vi "ROI entry-User ROI event-Analyse.vi"(8 "error in (no error)":errorcluster, 11 "Event Type":u32) -> (0 "error out":errorcluster, 2 "output cluster":T2 {"ROIs Info []"."FOV" min=1.0 max=10.0 step=1.0; "ROIs Info []"."Frame Size" min=1.0 max=10.0 step=1.0; "ROIs Info []"."Laser Power" min=1.0 max=10.0 step=0.10000000149011612; "ROIs Info []"."Rel. Resolution" min=1.0 max=10.0 step=1.0; "ROIs Info []"."POI Dwell time" min=1.0 max=10.0 step=0.10000000149011612; "ROIs Info []"."Zoom" min=1.0 max=10.0 step=0.10000000149011612; "Last Image Display Event info"."Tool" items=["None", "Selection Tool", "Point Tool", "Line Tool", "Rectangle Tool", "Oval Tool", "Polygon Tool", "ClosedFreehandTool", "Annulus Tool", "Rotated Rectangle Tool", "Zoom Tool", "Pan Tool", "Polyline Tool", "Freehand Tool"]; "Last Image Display Event info"."Type" items=["No Event"=0, "Click Event"=1, "Draw Event"=2, "Size Event"=4, "Scroll Event"=5, "Double Click Event"=8]})   [LabVIEW 2020]
uses:
  Typedefs/ROI Entry screen VI interface 1.ctl
  Typedefs/Last Image Display Event info.ctl
  Typedefs/ROI spec.ctl
  Typedefs/ROI ID Enum.ctl
  Typedefs/ROI info cluster.ctl
  ROI Entry screen/Globals/gl_ROI Entry UI globals.vi
panel:
  out "ROI info cluster (native format)":T1
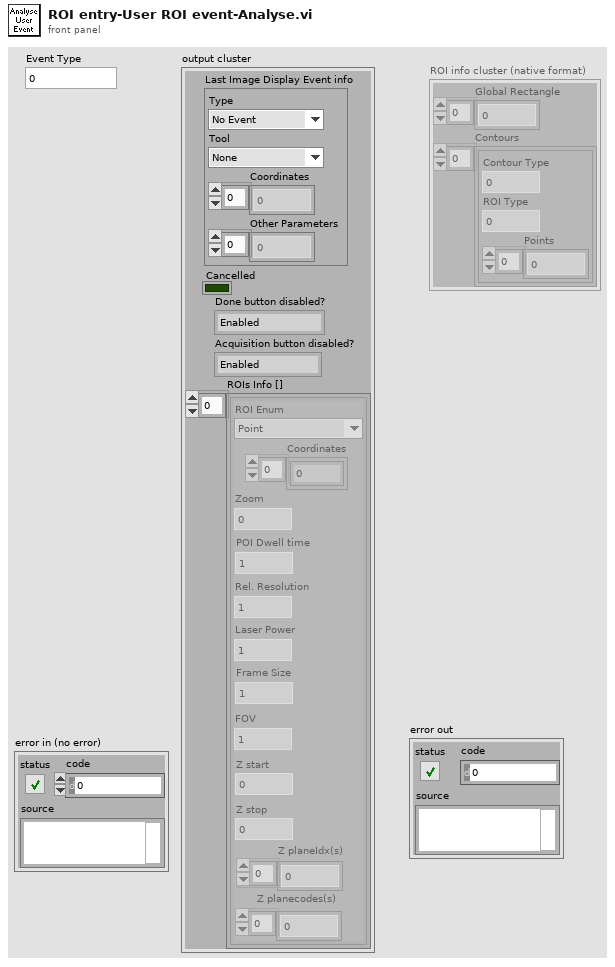
[diagram p1: front panel]
types:
  T1 = typedef "ROI info cluster.ctl" = cluster{"Global Rectangle":i32[], "Contours":cluster{"Contour Type":u32, "ROI Type":u32, "Points":i32[]}[]}
  T2 = typedef "ROI Entry screen VI interface 1.ctl" = cluster{"Last Image Display Event info":T3, "ROIs Info []":T4[], "Cancelled":bool, "Done button disabled?":enum8{"Enabled", "Disabled", "Disabled and Grayed Out"}, "Acquisition button disabled?":enum8{"Enabled", "Disabled", "Disabled and Grayed Out"}}
  T3 = typedef "Last Image Display Event info.ctl" = cluster{"Type":i32, "Tool":i32, "Coordinates":i32[], "Other Parameters":sgl[]}
  T4 = typedef "ROI spec.ctl" = cluster{"ROI Enum":T5, "Coordinates":i32[], "Zoom":dbl, "POI Dwell time":dbl, "Rel. Resolution":dbl, "Laser Power":dbl, "Frame Size":dbl, "FOV":dbl, "Z start":dbl, "Z stop":dbl, "Z planeIdx(s)":i32[], "Z planecodes(s)":u8[]}
  T5 = typedef "ROI ID Enum.ctl" = enum16{"Point", "MiniScan", "Comp. MiniScan", "Rectangle", "Comp. volume", "Arb. plane point", "None"}
  T6 = typedef "ROI entry screen ctrl refs cluster.ctl" = cluster{"Done button":refnum<vi>, "Imaging button":refnum<vi>, "Acquisition button":refnum<vi>, "Scan dwell time per pixel (us)":refnum<vi>, "# of planes":refnum<vi>, "Zoom Ctrl":refnum<vi>, "Equal size":refnum<vi>, "Channel":refnum<vi>, "Image Display":refnum<vi>, "Z-Plane Selector":refnum<vi>, "Number of lines left":refnum<vi>, "Z-stack folder path":refnum<vi>, "POI Density":refnum<vi>, "Arb Plane Entry":refnum<vi>, "Whole Plane":refnum<vi>, "Line Mode":refnum<vi>, "Clear Last":refnum<vi>, "Clear All":refnum<vi>, "Delete Lines":refnum<vi>, "Trial Length (sec)":refnum<vi>, "Palette Type":refnum<vi>, "Intensity slider":refnum<vi>, "# POI":refnum<vi>, "Max Z Proj":refnum<vi>, "Zplane ind":refnum<vi>, "Wavelength (nm)":refnum<vi>, "Number of Trials":refnum<vi>, "Funct stim.trig.enable":refnum<vi>, "Funct stim.trig.delay (s)":refnum<vi>, "Line Mode":refnum<vi>, "Step size (µm)":refnum<vi>, "ROI move mode":refnum<vi>, "Cool-down time (s)":refnum<vi>, "Enable cool-down time":refnum<vi>, "Motor Z ind. (um)":refnum<vi>, "AOL Z ind. (um)":refnum<vi>, "Load Reference Image":refnum<vi>, "Rel.  Res.":refnum<vi>, "ROI LIST":refnum<vi>, "Show All":refnum<vi>, "ROI Type":refnum<vi>, "Start Plane":refnum<vi>, "Stop Plane":refnum<vi>, "Offset ROI":refnum<vi>, "Tab Control":refnum<vi>, "Laser Power(%)":refnum<vi>, "Cycle rate":refnum<vi>, "FOV (Ind.)":refnum<vi>, "Frame Size (Ind.)":refnum<vi>, "Resolution (Ind.)":refnum<vi>, "Pixel Density (Ind)":refnum<vi>, "Laser Power (Ind.)":refnum<vi>, "Dwell Time (Ind.)":refnum<vi>, "Adj MC":refnum<vi>}
  T7 = enum8{"Enabled", "Disabled", "Disabled and Grayed Out"}
  T8 = typedef "ROI Z-stack settings info.ctl" = cluster{"Zoom":dbl, "POI Dwell time":dbl, "Rel. Res":dbl, "Laser Power %":dbl, "Frame Size":dbl, "FOV":dbl}
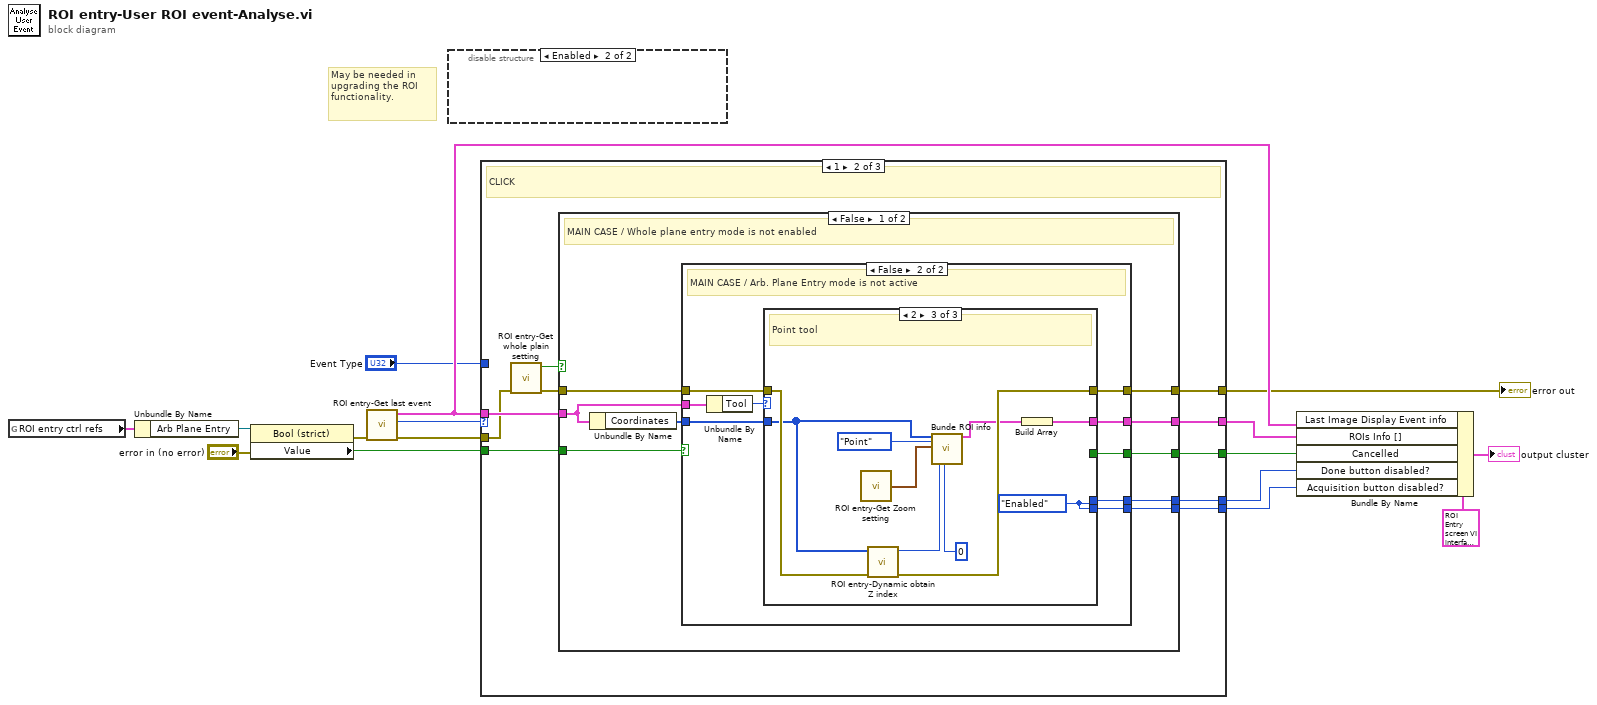
[diagram p0: block diagram]
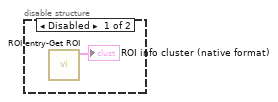
[diagram p2: hidden frame]
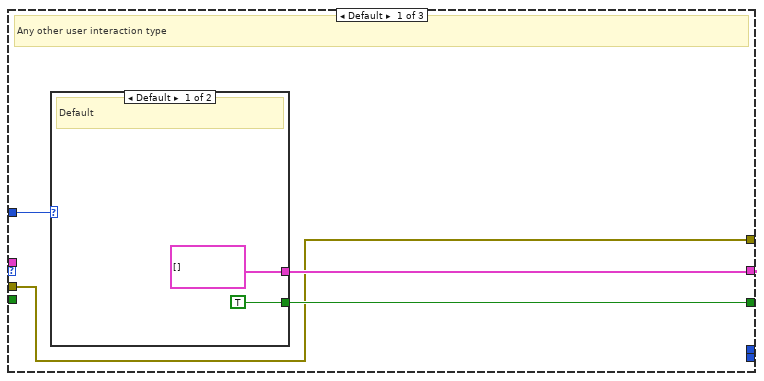
[diagram p3: hidden frame]
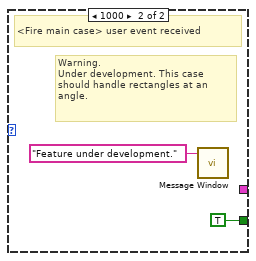
[diagram p4: hidden frame]
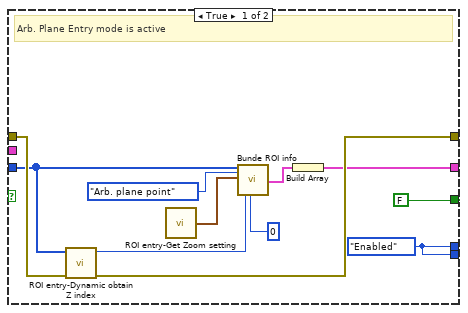
[diagram p5: hidden frame]
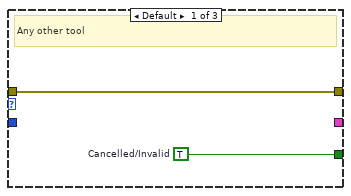
[diagram p6: hidden frame]
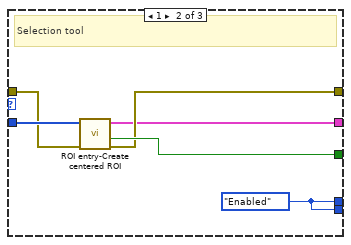
[diagram p7: hidden frame]
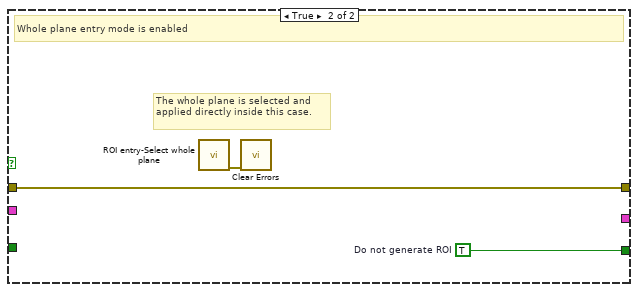
[diagram p8: hidden frame]
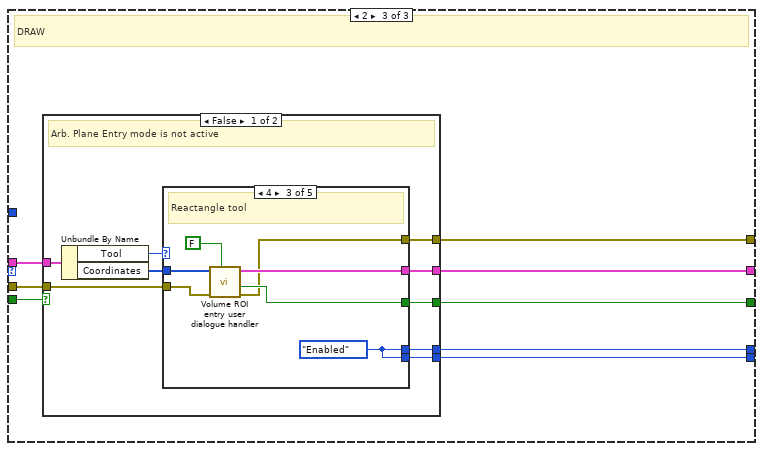
[diagram p9: hidden frame]
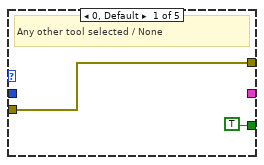
[diagram p10: hidden frame]
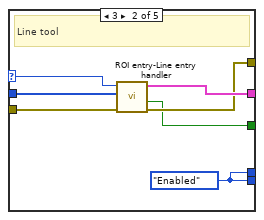
[diagram p11: hidden frame]
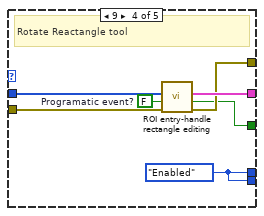
[diagram p12: hidden frame]
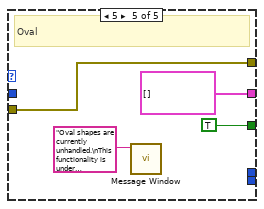
[diagram p13: hidden frame]
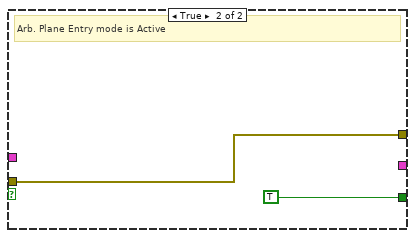
[diagram p14: hidden frame]
diagram:
  # "May be needed in upgrading the ROI functionality."
  n1 = global read "gl_ROI Entry UI globals.vi" "ROI entry ctrl refs"() -> (w15:T6)
  n2 = Unbundle By Name(w15) -> ("Arb Plane Entry"=w14:refnum<vi>)
  n3 = property class="Bool (strict)"(reference=w14, error in="error in (no error)") -> (error out=w4:errorcluster, "Value"=w16:bool)  [unwired: 1 out]
  n4 = call "ROI entry-Get last event.vi"("error in (no error)"=w4) -> ("error out"=w2:errorcluster, "Type"=w6:i32, "Last Image Display Event info"=w13:T3)  [unwired: 8 in]
  n5 = disable-structure shown="Enabled" {
    frame Disabled {
      n6 = call "ROI entry-Get ROI.vi"() -> ("ROI info cluster (native format)"=→"ROI info cluster (native format)":T1)  [unwired: 10 in, 1 out]
    }
    frame Enabled {
    }
  }
  n7 = case shown="1" w6 {
    tunnel: [w20 w26 w93] -> w7
    tunnel: [w19 w35 w92] -> w11
    tunnel: [_ w34 w91] -> w8
    tunnel: [_ w33 w90] -> w9
    tunnel: "Event Type" -> [w21 _ _]
    tunnel: w16 -> [_ w32 w89]
    tunnel: w13 -> [_ w31 w88]
    tunnel: w2 -> [w18 w29 w86]
    tunnel: [w18 w27 w87] -> w1
    frame Default {
      # "Any other user interaction type"
      n8 = case shown="Default" w21 {
        tunnel: [T4[] [] ("ROIs Info []") _] -> w20
        tunnel: [TRUE TRUE ("Cancelled")] -> w19
        frame Default {
          # "Default"
        }
        frame 1000 {
          # "Warning.\nUnder development. This case should handle rectangles at an angle."
          # "<Fire main case> user event received"
          n9 = call "Message Window.vi"("Message string"="Feature under development." ("message")) -> ()  [unwired: 10 in, 1 out]
        }
      }
    }
    frame 1 {
      # "CLICK"
      n10 = call "ROI entry-Get whole plain setting.vi"("error in (no error)"=w29) -> ("error out"=w28:errorcluster, "\"Whole plain?\" value"=w30:bool)  [unwired: 9 in]
      n11 = case shown="False" w30 {
        tunnel: [w44 w85] -> w35
        tunnel: [w43 _] -> w34
        tunnel: [w42 _] -> w33
        tunnel: w32 -> [w41 _]
        tunnel: w31 -> [w39 _]
        tunnel: w28 -> [w36 w83]
        tunnel: [w37 w83] -> w27
        tunnel: [w38 _] -> w26
        frame False {
          # "MAIN CASE / Whole plane entry mode is not enabled"
          n12 = Unbundle By Name(w39) -> ("Coordinates"=w40:i32[])
          n13 = case shown="False" w41 {
            tunnel: w40 -> [w51 w64]
            tunnel: [FALSE ("Do not generate ROI") w63] -> w44
            tunnel: [w55 w62] -> w43
            tunnel: [w55 w61] -> w42
            tunnel: w39 -> [_ w60]
            tunnel: w36 -> [w53 w58]
            tunnel: [w52 w57] -> w37
            tunnel: [w50 w56] -> w38
            frame True {
              w55 = T7."Enabled" ("Disabled")
              # "Arb. Plane Entry mode is active"
              n14 = call "ROI entry-Dynamic obtain Z index.vi"("error in (no error)"=w53, "Coordinates"=w51) -> ("error out"=w52:errorcluster, "Z-plane selector (index)"=w47:i32)  [unwired: 8 in]
              n15 = call "ROI entry-Get Zoom setting.vi"() -> ("AOLZ Settings"=w45:T8)  [unwired: 7 in, 8 out]
              n16 = call "Bunde ROI info.vi"("ROI Coordinates"=w51, "ROI Enum"=ROI_ID_Enum."Arb. plane point", "Z stack Settings"=w45, "ZplaneIndex"=w47, "Zplanecode"=u8 0) -> ("ROI Info"=w49:T4)  [unwired: 14 in]
              n17 = Build Array(w49) -> (w50:T4[])
            }
            frame False {
              # "MAIN CASE / Arb. Plane Entry mode is not active"
              n18 = Unbundle By Name(w60) -> ("Tool"=w59:i32)
              n19 = case shown="2" w59 {
                tunnel: w64 -> [_ w71 w76]
                tunnel: [w66 w69 _] -> w63
                tunnel: [_ w72 w82] -> w62
                tunnel: [_ w72 w82] -> w61
                tunnel: w58 -> [w65 w70 w80]
                tunnel: [w65 w68 w81] -> w57
                tunnel: [_ w67 w79] -> w56
                frame Default {
                  w66 = TRUE  # Cancelled/Invalid
                  # "Any other tool"
                }
                frame 1 {
                  w72 = T7."Enabled" ("Disabled")
                  # "Selection tool"
                  n20 = call "ROI entry-Create centered ROI.vi"("error in (no error)"=w70, "Coordinates"=w71) -> ("error out"=w68:errorcluster, "Do not generate ROI"=w69:bool, "ROIs Info []"=w67:T4[])  [unwired: 7 in]
                }
                frame 2 {
                  w82 = T7."Enabled" ("Disabled")
                  # "Point tool"
                  n21 = call "ROI entry-Get Zoom setting.vi"() -> ("AOLZ Settings"=w73:T8)  [unwired: 7 in, 8 out]
                  n22 = call "ROI entry-Dynamic obtain Z index.vi"("error in (no error)"=w80, "Coordinates"=w76) -> ("error out"=w81:errorcluster, "Z-plane selector (index)"=w74:i32)  [unwired: 8 in]
                  n23 = call "Bunde ROI info.vi"("ROI Coordinates"=w76, "ROI Enum"=ROI_ID_Enum."Point", "Z stack Settings"=w73, "ZplaneIndex"=w74, "Zplanecode"=u8 0) -> ("ROI Info"=w78:T4)  [unwired: 14 in]
                  n24 = Build Array(w78) -> (w79:T4[])
                }
              }
            }
          }
        }
        frame True {
          w85 = TRUE  # Do not generate ROI
          # "The whole plane is selected and applied directly inside this case."
          # "Whole plane entry mode is enabled"
          n25 = call "ROI entry-Select whole plane.vi"() -> ("error IO"=w84:errorcluster)  [unwired: 11 in]
          n26 = call <vilib>:"Clear Errors.vi"("error in (no error)"=w84) -> ()  [unwired: 5 in, 2 out]
        }
      }
    }
    frame 2 {
      # "DRAW"
      n27 = case shown="False" w89 {
        tunnel: [w102 _] -> w93
        tunnel: [w101 TRUE ("Cancelled")] -> w92
        tunnel: [w100 _] -> w91
        tunnel: [w99 _] -> w90
        tunnel: w88 -> [w98 _]
        tunnel: [w94 w130] -> w87
        tunnel: w86 -> [w95 w130]
        frame False {
          # "Arb. Plane Entry mode is not active"
          n28 = Unbundle By Name(w98) -> ("Tool"=w97:i32, "Coordinates"=w96:i32[])
          n29 = case shown="4" w97 {
            selector: w97 -> [_ w108 _ _ _]
            tunnel: w96 -> [_ w109 w116 w123 _]
            tunnel: [_ w111 w118 w125 T4[] [] ("ROIs Info []")] -> w102
            tunnel: [TRUE w105 w114 w119 TRUE ("Cancelled")] -> w101
            tunnel: [_ w110 w117 w124 _] -> w100
            tunnel: [_ w110 w117 w124 _] -> w99
            tunnel: [w103 w107 w113 w120 w127] -> w94
            tunnel: w95 -> [w103 w106 w115 w121 w127]
            frame 0, Default {
              # "Any other tool selected / None"
            }
            frame 3 {
              w110 = T7."Enabled" ("Disabled")
              # "Line tool"
              n30 = call "ROI entry-Line entry handler.vi"("error in (no error)"=w106, "Coordinates"=w109, "Tool"=w108) -> ("error out"=w107:errorcluster, "Do not generate line ROI"=w105:bool, "Array"=w111:T4[])  [unwired: 6 in]
            }
            frame 4 {
              w117 = T7."Enabled" ("Disabled")
              # "Reactangle tool"
              n31 = call "Volume ROI entry user dialogue handler.vi"("Center around clicked pixel (F)"=FALSE, "error in (no error)"=w115, "New coordinates"=w116) -> ("error IO"=w113:errorcluster, "Cancelled"=w114:bool, "ROIs Info []"=w118:T4[])  [unwired: 6 in]
            }
            frame 9 {
              w122 = FALSE  # Programatic event?
              w124 = T7."Enabled" ("Disabled")
              # "Rotate Reactangle tool"
              n32 = call "ROI entry-handle rectangle editing.vi"("error in (no error)"=w121, "Programatic event?"=w122, "Coordinates"=w123) -> ("error IO"=w120:errorcluster, "Cancelled"=w119:bool, "ROIs Info []"=w125:T4[])  [unwired: 6 in]
            }
            frame 5 {
              # "Oval"
              n33 = call "Message Window.vi"("Message string"="Oval shapes are currently unhandled.\nThis functionality is under development." ("message")) -> ()  [unwired: 10 in, 1 out]
            }
          }
        }
        frame True {
          # "Arb. Plane Entry mode is Active"
        }
      }
    }
  }
  "error out" <- w1
  n34 = Bundle By Name(cluster=T2 {"Last Image Display Event info"={"Type"=0, "Tool"=0, "Coordinates"=[], "Other Parameters"=[]}, "ROIs Info []"=[], "Cancelled"=FALSE, "Done button disabled?"=enum."Enabled", "Acquisition button disabled?"=enum."Enabled"} ("output cluster"), "Last Image Display Event info"=w13, "ROIs Info []"=w7, "Cancelled"=w11, "Done button disabled?"=w8, "Acquisition button disabled?"=w9) -> (→"output cluster":T2)
